vi "Create.vi"(9 "Alias":string, 10 "Actor":refnum<class "Actor.lvclass">, 11 "Ex Queue Actor in":refnum<class "Ex Queue Actor.lvclass">) -> (3 "Ex Queue Actor out":refnum<class "Ex Queue Actor.lvclass">)   [LabVIEW 2021, in "Ex Queue Actor.lvlib" / "Ex Queue Actor.lvclass"]
uses:
  Ex Queue Actor.lvclass
  Actor/Actor/Actor.lvclass
  Ex Queue Actor.lvclass/Ex Queue Actor.ctl
  Actor/Queue Actor/Queue Actor.lvclass
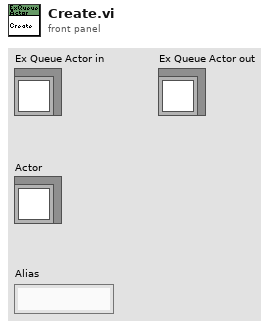
[diagram p1: front panel]
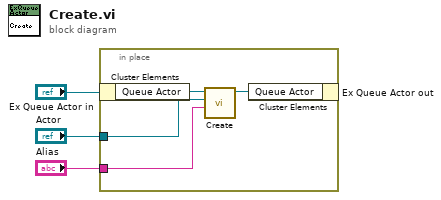
[diagram p0: block diagram]
diagram:
  n1 = in-place {
    in-place-border: "Actor" -> [w5]
    in-place-border: "Alias" -> [w6]
    n2 = in-place-cluster #1("Ex Queue Actor in") -> ("Queue Actor"=w7:refnum<class "Queue Actor.lvclass">)
    n3 = call-dynamic "Create.vi"("Alias"=w6, "Actor"=w5, "Create in"=w7) -> ("Create out"=w8:refnum<class "Queue Actor.lvclass">)  [unwired: 8 in]
    n4 = in-place-cluster #1("Queue Actor"=w8) -> (→"Ex Queue Actor out":refnum<class "Ex Queue Actor.lvclass">)
  }
